vi "DAQNavi Read (Digital 1D U8 1Chan NSamp).vi"(8 "error in (no error)":errorcluster, 9 "timeout":dbl=10.0, 10 "number of samples per channel to read":u32=1000, 11 "task in":i32) -> (0 "error out":errorcluster, 2 "data":u8[](array[numeric]), 3 "task out":i32)   [LabVIEW 2020]
uses:
  DAQNavi_LV.dll
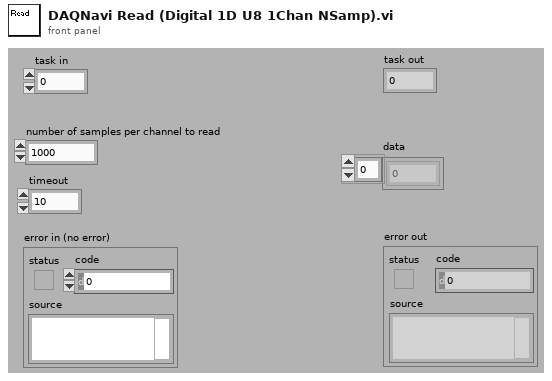
[diagram p1: front panel]
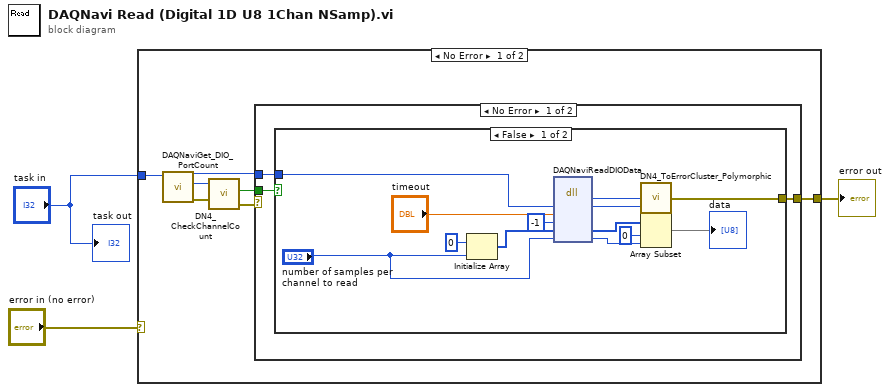
[diagram p0: block diagram]
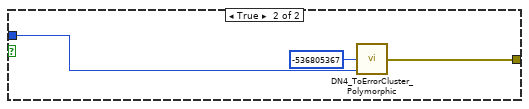
[diagram p2: hidden frame]
diagram:
  n1 = case shown="No Error" "error in (no error)" {
    selector: "error in (no error)" -> [_ w31]
    tunnel: "task in" -> [w10 _]
    tunnel: [w4 w31] -> w1
    frame No Error {
      n2 = call "DAQNaviGet_DIO_PortCount.vi"("task in"=w10) -> ("error out"=w9:errorcluster, "port count"=w8:i32, "task out"=w5:i32)  [unwired: 1 in, 7 out]
      n3 = call "DN4_CheckChannelCount.vi"("error out"=w9, "channel count"=w8) -> ("error IO"=w7:errorcluster, "greater than 1?"=w6:bool)  [unwired: 2 out]
      n4 = case shown="No Error" w7 {
        selector: w7 -> [_ w30]
        tunnel: [w13 w30] -> w4
        tunnel: w6 -> [w12 _]
        tunnel: w5 -> [w11 _]
        frame No Error {
          n5 = case shown="False" w12 {
            tunnel: [w25 w28] -> w13
            tunnel: w11 -> [w24 w27]
            frame False {
              n6 = Initialize Array(u8 0 ("element"), "number of samples per channel to read") -> (w16:u8[])
              n7 = dll-call lib="DAQNavi_LV.dll" fn="DAQNaviReadDIOData"("taskID"=w24, "timeout"="timeout", "portBit"=-1, "portData"=w16, "samples"="number of samples per channel to read") -> ("return type"=w26:i32, "taskID"=w15:i32, "portData"=w22:u8[], "samples"=w20:u32)  [unwired: 5 in, 2 out]
              n8 = call "DN4_ToErrorCluster_Polymorphic.vi"("task id"=w15, "error code"=w26) -> ("error out"=w25:errorcluster)  [unwired: 3 out]
              n9 = Array Subset(array=w22, index=0, length=w20) -> (→"data":u8[])
            }
            frame True {
              n10 = call "DN4_ToErrorCluster_Polymorphic.vi"("task id"=w27, "error code"=-536805367 ("error code (0)")) -> ("error out"=w28:errorcluster)  [unwired: 3 out]
            }
          }
        }
        frame Error {
        }
      }
    }
    frame Error {
    }
  }
  "error out" <- w1
  "task out" <- "task in"
